vi "Get Proximity.vi"(8 "error in (no error)":errorcluster, 11 "ColorSensorDevRef":T1={"I2CDevRef"={"DevStatus"={"status"=FALSE, "code"=0, "source"=""}, "Device Address"=0, "Handle"=0, "I2C Bus"=enum."Invalid"}} {"I2CDevRef"."Device Address" format="%.0x"}) -> (0 "error out":errorcluster, 2 "Proximity":u16, 3 "ColorSensorDevRef out":T1={"I2CDevRef"={"DevStatus"={"status"=FALSE, "code"=0, "source"=""}, "Device Address"=0, "Handle"=0, "I2C Bus"=enum."Invalid"}} {"I2CDevRef"."Device Address" format="%.0x"})   [LabVIEW 2018, in "ColorSensor.lvlib"]
uses:
  ColorSensor.lvlib
  ColorSensorDevRef.ctl
  <vilib>/Rock Robotics/WPI/I2C/WPI_I2CDevRef.ctl
  <vilib>/Rock Robotics/SystemInterfaces/i2clib/i2c_bus.ctl
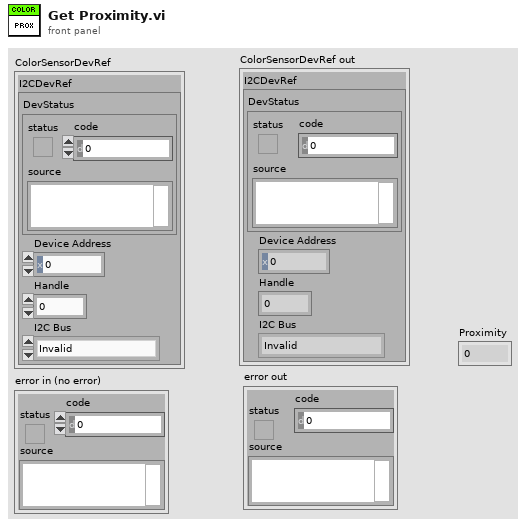
[diagram p1: front panel]
types:
  T1 = typedef "ColorSensor.lvlib/ColorSensorDevRef.ctl" = cluster{"I2CDevRef":T2}
  T2 = typedef "WPI_I2CDevRef.ctl" = cluster{"DevStatus":errorcluster, "Device Address":u8, "Handle":i32, "I2C Bus":T3}
  T3 = typedef "i2c_bus.ctl" = enum16{"I2C On-Board", "I2C MXP", "Invalid"}
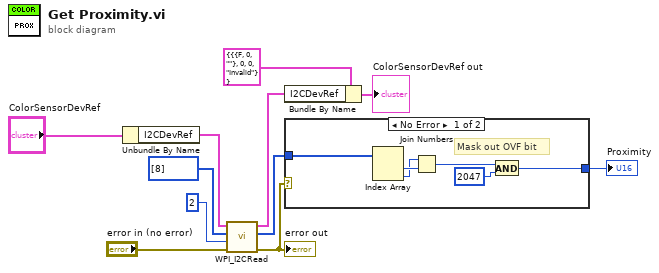
[diagram p0: block diagram]
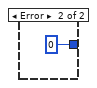
[diagram p2: hidden frame]
diagram:
  n1 = Unbundle By Name("ColorSensorDevRef") -> ("I2CDevRef"=w10:T2)
  n2 = call <vilib>:"WPI_I2CRead.vi"("error in (no error)"="error in (no error)", "I2CBytesToRead"=u8 2, "I2CRegister"=u8[] [8], "I2CDevRef"=w10) -> ("error out"=w6:errorcluster, "Data Out"=w5:u8[], "I2CDevRef"=w2:T2)  [unwired: 5 in]
  "error out" <- w6
  n3 = Bundle By Name(cluster=T1 {"I2CDevRef"={"DevStatus"={"status"=FALSE, "code"=0, "source"=""}, "Device Address"=0, "Handle"=0, "I2C Bus"=enum."Invalid"}} ("ColorSensorDevRef"), "I2CDevRef"=w2) -> (→"ColorSensorDevRef out":T1)
  n4 = case shown="No Error" w6 {
    tunnel: w5 -> [w17 _]
    tunnel: [w12 u16 0] -> w4
    frame No Error {
      # "Mask out OVF bit"
      n5 = Index Array(array=w17) -> (element #1=w16:u8, element #2=w15:u8)  [unwired: 2 in]
      n6 = Join Numbers(hi=w15, lo=w16) -> ((hi.lo)=w14:u16)
      n7 = And(x=w14, y=u16 2047) -> (x .and. y?=w12:u16)
    }
    frame Error {
    }
  }
  "Proximity" <- w4
